vi "Ejemplo_clase6.vi"() -> ()   [LabVIEW 2020]
panel:
  out "Array":dbl[](array[numeric])
  in  "Numeric":i32
  in  "Lim Min T":dbl
  in  "Lim Max T":dbl
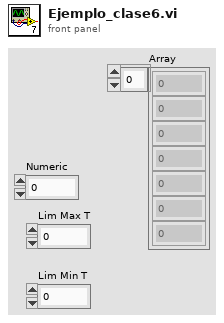
[diagram p1: front panel]
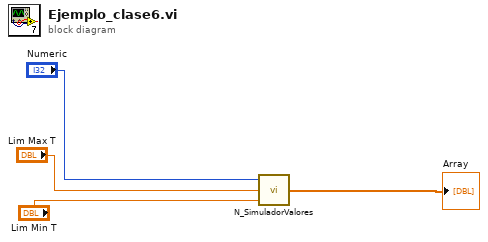
[diagram p0: block diagram]
diagram:
  n1 = call "N_SimuladorValores.vi"("Lim Max T"="Lim Min T", "Lim Min T"="Lim Max T", "Numeric"="Numeric") -> ("Array"=→"Array":dbl[])
